vi "Measurement Plugin Path - Single Converter.vi"(11 "error in":errorcluster) -> (0 "measurement ui lib":path, 1 "run service":path, 2 "measurement ui":path, 3 "instrumentstudio folder":path, 4 "new code module":path, 5 "set default value":path, 6 "wrapper path":path, 8 "result control":path, 10 "input controls":path, 12 "library":path, 13 "type specialization":path, 14 "logic vi path":path, 15 "error out":errorcluster)   [LabVIEW 2021, in "Path Functions.lvlib"]
uses:
  Path Functions.lvlib
  Converter Reusables/Converter Reusables.lvlib
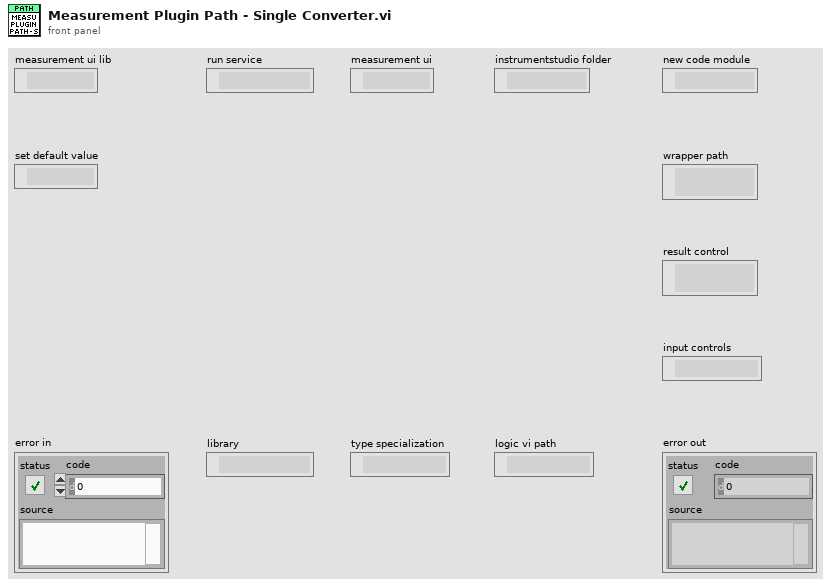
[diagram p1: front panel]
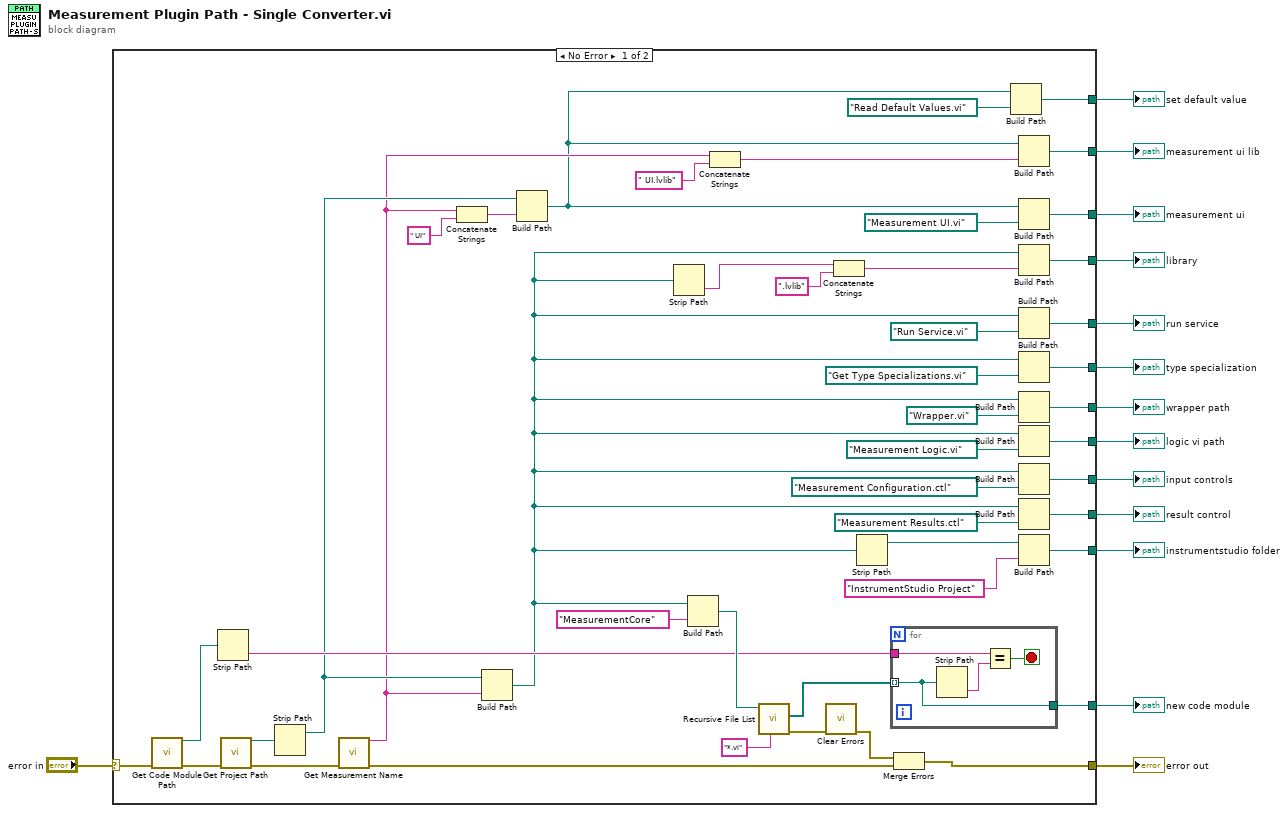
[diagram p0: block diagram]
diagram:
  n1 = case shown="No Error" "error in" {
    selector: "error in" -> [w44 w66]
    tunnel: [w61 _] -> w14
    tunnel: [w60 _] -> w13
    tunnel: [w59 _] -> w12
    tunnel: [w58 _] -> w11
    tunnel: [w52 _] -> w10
    tunnel: [w51 _] -> w9
    tunnel: [w49 _] -> w8
    tunnel: [w46 _] -> w7
    tunnel: [w40 _] -> w6
    tunnel: [w30 w66] -> w5
    tunnel: [w17 _] -> w4
    tunnel: [w22 _] -> w3
    tunnel: [w21 _] -> w2
    frame No Error {
      n2 = call "Get Code Module Path.vi"("error in"=w44) -> ("code module out"=w42:path, "error out"=w43:errorcluster)  [unwired: 13 in]
      n3 = Strip Path(path=w42) -> (name=w32:string)  [unwired: 1 out]
      n4 = call "Get Project Path.vi"("error in"=w43) -> ("project path out"=w16:path, "error out"=w45:errorcluster)  [unwired: 13 in]
      n5 = Strip Path(path=w16) -> (stripped path=w28:path)  [unwired: 1 out]
      n6 = call "Get Measurement Name.vi"("error in"=w45) -> ("name out"=w23:string, "error out"=w31:errorcluster)  [unwired: 13 in]
      n7 = Concatenate Strings(w23, " UI" ("string")) -> (w26:string)
      n8 = Build Path(base path=w28, name or relative path=w23) -> (appended path=w29:path)
      n9 = Build Path(base path=w28, name or relative path=w26) -> (appended path=w20:path)
      n10 = Strip Path(path=w29) -> (name=w41:string)  [unwired: 1 out]
      n11 = Build Path(base path=w29, name or relative path="MeasurementCore" ("string")) -> (appended path=w35:path)
      n12 = Concatenate Strings(w23, " UI.lvlib" ("string")) -> (w24:string)
      n13 = call <vilib>:"Recursive File List.vi"("pattern"="*.vi", "Folder Path"=w35) -> ("error out"=w34:errorcluster, "All Files in Dir"=w36:path[])  [unwired: 5 in, 3 out]
      n14 = call <vilib>:"Clear Errors.vi"("error in (no error)"=w34) -> ("error out"=w33:errorcluster)  [unwired: 5 in, 1 out]
      n15 = Concatenate Strings(w41, ".lvlib" ("string")) -> (w39:string)
      n16 = Strip Path(path=w29) -> (stripped path=w48:path)  [unwired: 1 out]
      n17 = for {
        tunnel: w36 -> [w63] mode=indexing
        tunnel: w32 -> [w65]
        tunnel: [w63] -> w17
        stop <- w62 stop-if-true
        n18 = Strip Path(path=w63) -> (name=w64:string)  [unwired: 1 out]
        n19 = Equal?(x=w65, y=w64) -> (x = y?=w62:bool)
      }
      n20 = Merge Errors(w33, w31) -> (w30:errorcluster)
      n21 = Build Path(base path=w20, name or relative path=path "Read Default Values.vi") -> (appended path=w21:path)
      n22 = Build Path(base path=w20, name or relative path=w24) -> (appended path=w22:path)
      n23 = Build Path(base path=w20, name or relative path=path "Measurement UI.vi") -> (appended path=w52:path)
      n24 = Build Path(base path=w29, name or relative path=w39) -> (appended path=w40:path)
      n25 = Build Path(base path=w29, name or relative path=path "Run Service.vi") -> (appended path=w46:path)
      n26 = Build Path(base path=w29, name or relative path=path "Get Type Specializations.vi") -> (appended path=w51:path)
      n27 = Build Path(base path=w29, name or relative path=path "Wrapper.vi") -> (appended path=w61:path)
      n28 = Build Path(base path=w29, name or relative path=path "Measurement Logic.vi") -> (appended path=w60:path)
      n29 = Build Path(base path=w29, name or relative path=path "Measurement Configuration.ctl") -> (appended path=w59:path)
      n30 = Build Path(base path=w29, name or relative path=path "Measurement Results.ctl") -> (appended path=w58:path)
      n31 = Build Path(base path=w48, name or relative path="InstrumentStudio Project" ("string")) -> (appended path=w49:path)
    }
    frame Error {
    }
  }
  "error out" <- w5
  "new code module" <- w4
  "wrapper path" <- w14
  "logic vi path" <- w13
  "input controls" <- w12
  "result control" <- w11
  "instrumentstudio folder" <- w8
  "measurement ui" <- w10
  "type specialization" <- w9
  "run service" <- w7
  "library" <- w6
  "measurement ui lib" <- w3
  "set default value" <- w2
